vi "Wait on signal.vi"(8 "error in (no error)":errorcluster, 10 "Seconds to wait":i32, 11 "Signaller in":refnum<class "Signaller.lvclass">) -> (0 "error out":errorcluster, 3 "Signaller out":refnum<class "Signaller.lvclass">)   [LabVIEW 2018, in "Signaller.lvclass"]
uses:
  Signaller.lvclass
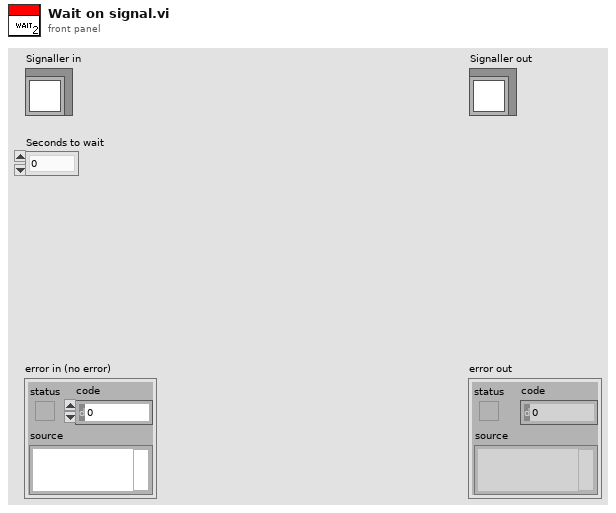
[diagram p1: front panel]
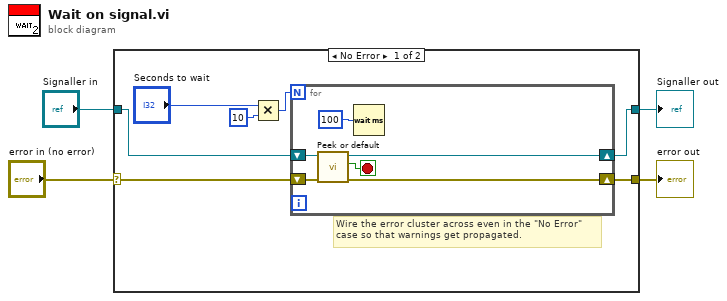
[diagram p0: block diagram]
diagram:
  n1 = case shown="No Error" "error in (no error)" {
    selector: "error in (no error)" -> [w6 w19]
    tunnel: [w5 w19] -> w3
    tunnel: [w7 w18] -> w1
    tunnel: "Signaller in" -> [w8 w18]
    frame No Error {
      # "Wire the error cluster across even in the \"No Error\"\ncase so that warnings get propagated."
      n2 = Multiply(x="Seconds to wait", y=10) -> (x*y=w9:i32)
      n3 = for {
        N: w9 -> [_]
        shift-right: [w16] -> w7
        shift-left: w8 -> [w17]
        shift-right: [w14] -> w5
        shift-left: w6 -> [w13]
        stop <- w15 stop-if-true
        n4 = call "Peek or default.vi"("error in (no error)"=w13, "Signaller in"=w17) -> ("error out"=w14:errorcluster, "Has signal?"=w15:bool, "Signaller out"=w16:refnum<class "Signaller.lvclass">)  [unwired: 7 in]
        n5 = Wait (ms)(milliseconds to wait=u32 100) -> ()  [unwired: 1 out]
      }
    }
    frame Error {
    }
  }
  "error out" <- w3
  "Signaller out" <- w1
